vi "Set Temp Ramp Rate--Method.vi"(8 "error in (no error)":errorcluster, 10 "Temp Ramp Data":T1, 11 "Simulated Thermal Process Controller in":refnum<class "Simulated Thermal Process Controller.lvclass">) -> (0 "error out":errorcluster, 3 "Simulated Thermal Process Controller out":refnum<class "Simulated Thermal Process Controller.lvclass">)   [LabVIEW 2024, in "Simulated Thermal Process Controller.lvclass"]
uses:
  Simulated Thermal Process Controller.lvclass
  Process Controller/Controls/Temp Ramp Rate Data--Cluster.ctl
  Process Controller/Controls/Temperature Units--Enum.ctl
  Process Controller/Controls/Rate Units--Enum.ctl
  Simulated Thermal Process Controller.lvclass/Simulated Thermal Process Controller.ctl
  Process Controller/_Thermal Process Controller.lvclass
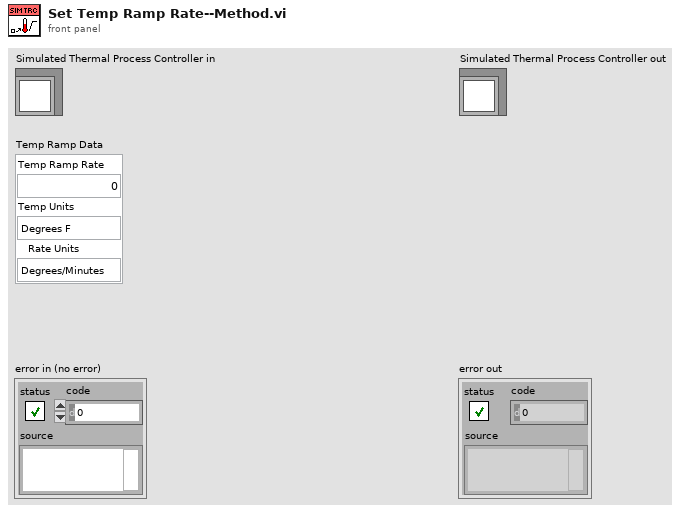
[diagram p1: front panel]
types:
  T1 = typedef "_Thermal Process Controller.lvclass/Temp Ramp Rate Data--Cluster.ctl" = cluster{"Temp Ramp Rate":dbl, "Temp Units":T2, "Rate Units":T3}
  T2 = typedef "_Thermal Process Controller.lvclass/Temperature Units--Enum.ctl" = enum16{"Degrees F", "Degrees C", "Degrees K"}
  T3 = typedef "_Thermal Process Controller.lvclass/Rate Units--Enum.ctl" = enum16{"Degrees/Minutes", "Degrees/Hours"}
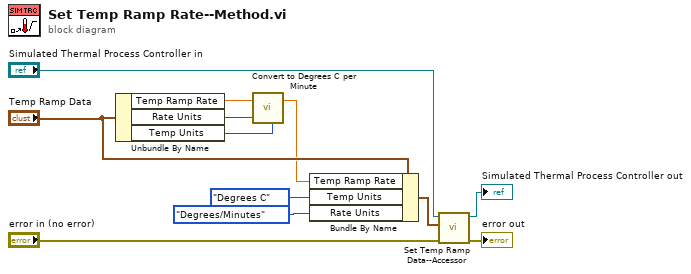
[diagram p0: block diagram]
diagram:
  n1 = Unbundle By Name("Temp Ramp Data") -> ("Temp Ramp Rate"=w8:dbl, "Rate Units"=w1:T3, "Temp Units"=w2:T2)
  n2 = call "Convert to Degrees C per Minute.vi"("Rate In"=w8, "Rate Units"=w1, "Temp Units"=w2) -> ("Rate Out"=w6:dbl)  [unwired: 4 in]
  n3 = Bundle By Name(cluster="Temp Ramp Data", "Temp Ramp Rate"=w6, "Temp Units"=Temperature_Units--Enum."Degrees C", "Rate Units"=Rate_Units--Enum."Degrees/Minutes") -> (w3:T1)
  n4 = call "Set Temp Ramp Data--Accessor.vi"("error in (no error)"="error in (no error)", "Temp Ramp Data"=w3, "Simulated Thermal Process Controller in"="Simulated Thermal Process Controller in") -> ("error out"=→"error out":errorcluster, "Simulated Thermal Process Controller out"=→"Simulated Thermal Process Controller out":refnum<class "Simulated Thermal Process Controller.lvclass">)  [unwired: 7 in]
